vi "Close FP if in LabVIEW Dir.vi"(7 "VI Refnum":refnum<vi>, 8 "Error in":errorcluster caption="Error in (no error)") -> (0 "Error out":errorcluster)   [LabVIEW 2017, in "csm-ui-support.lvlib"]
uses:
  csm-ui-support.lvlib
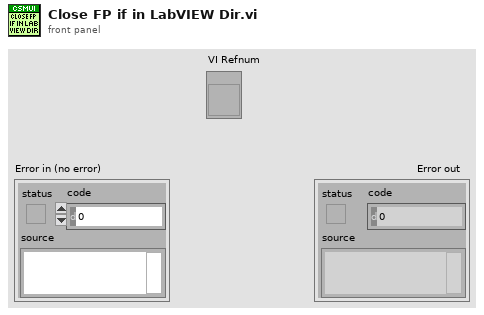
[diagram p1: front panel]
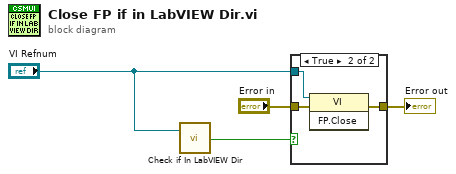
[diagram p0: block diagram]
diagram:
  n1 = call "Check if In LabVIEW Dir.vi"("VI Refnum"="VI Refnum") -> ("Boolean"=w4:bool)  [unwired: 1 in]
  n2 = case shown="True" w4 {
    tunnel: [w5 w8] -> w3
    tunnel: "Error in" -> [w5 w7]
    tunnel: "VI Refnum" -> [_ w6]
    frame False {
    }
    frame True {
      n3 = invoke class="VI" method="FP.Close"(reference=w6, error in=w7) -> (error out=w8:errorcluster)  [unwired: 1 in, 2 out]
    }
  }
  "Error out" <- w3
